vi "Test - cameraV1 - Cam Image Response 2.vi"(8 "error in":errorcluster, 11 "Module ID":i32) -> (0 "error out":errorcluster, 3 "Pass":bool)   [LabVIEW 2024]
doc: "_____\nCreated using DQMH Framework: Event Scripter 7.1.0.1503."
uses:
  Libraries/cameraV1/cameraV1.lvlib
panel:
  out "serial":string
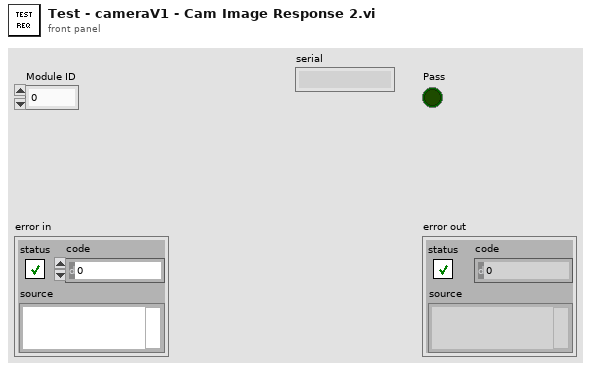
[diagram p1: front panel]
types:
  T1 = typedef "cameraV1.lvlib/Broadcast Events--cluster.ctl" = cluster{"Module Did Init":refnum<user-event>, "Status Updated":refnum<user-event>, "Error Reported":refnum<user-event>, "Module Did Stop":refnum<user-event>, "Update Module Execution Status":refnum<user-event>, "out reselt":refnum<user-event>}
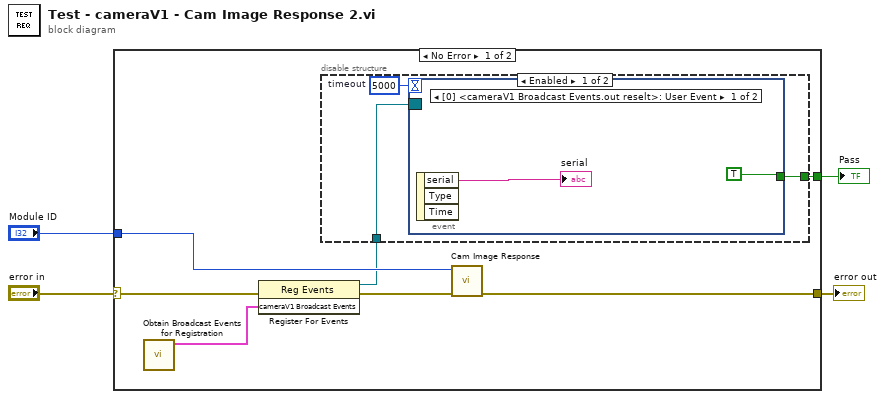
[diagram p0: block diagram]
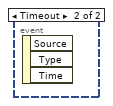
[diagram p2: hidden frame]
diagram:
  n1 = case shown="No Error" "error in" {
    selector: "error in" -> [w11 w17]
    tunnel: [w10 w17] -> w3
    tunnel: "Module ID" -> [w9 _]
    tunnel: [w5 _] -> w1
    frame No Error {
      n2 = call "Obtain Broadcast Events for Registration.vi"() -> ("cameraV1 Broadcast Events"=w7:T1)  [unwired: 9 in, 2 out]
      n3 = register-events(error in=w11, w7) -> (reference out=w6:refnum<event-registration>, error out=w8:errorcluster)  [unwired: 1 in]
      n4 = disable-structure shown="Enabled" {
        disable-tunnel: w6 -> [w14 _]
        disable-tunnel: [w12 _] -> w5
        frame Enabled {
          w13 = 5000  # timeout
          n5 = event shown="[0] <cameraV1 Broadcast Events.out reselt>: User Event" {
            selector: w14 -> [_ _]
            dyn-events: _ -> [_ _]
            timeout: w13 -> [_ _]
            tunnel: [TRUE _] -> w12
            event User Event {
              n6 = event-data() -> ("serial"=→"serial":string)  [unwired: 1 in, 2 out]
            }
            event Timeout {
              n7 = event-data() -> ()  [unwired: 1 in, 3 out]
            }
          }
        }
        frame Disabled {
        }
      }
      n8 = call "Cam Image Response.vi"("error in"=w8, "Module ID"=w9) -> ("error out"=w10:errorcluster)  [unwired: 9 in]
    }
    frame Error {
    }
  }
  "error out" <- w3
  "Pass" <- w1
